vi "Rohde & Schwarz VNA Set Sweep Type.vi"(6 "Channel":i8=1 min=1 max=99 step=1, 7 "Rohde & Schwarz VNA":T1, 8 "error in (no error)":errorcluster, 10 "Sweep Type":T2, 11 "VISA Resource Name":refnum<visa-resource-name>) -> (0 "error out":errorcluster, 3 "dup VISA Resource Name":refnum<visa-resource-name>)   [LabVIEW 2011]
doc: "This VI for the HP8753B is used to set the meausurement format."
uses:
  TypeDefs/Rohde & Schwarz VNA Sweep Type.ctl
  TypeDefs/Rohde & Schwarz VNA Instrument Info.ctl
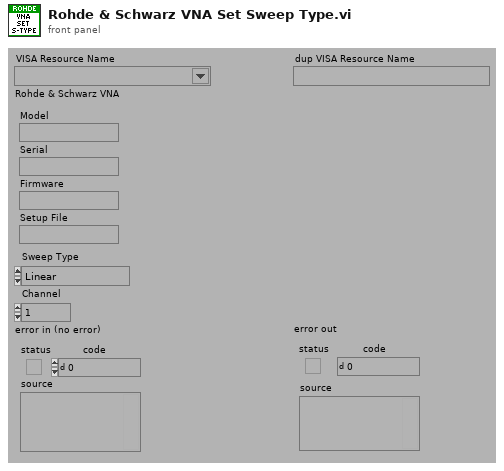
[diagram p1: front panel]
types:
  T1 = typedef "Rohde & Schwarz VNA Instrument Info.ctl" = cluster{"Model":string, "Serial":string, "Firmware":string, "Setup File":string}
  T2 = typedef "Rohde & Schwarz VNA Sweep Type.ctl" = enum32{"Linear", "Logarithmic", "Segmented", "Power", "Time", "CW"}
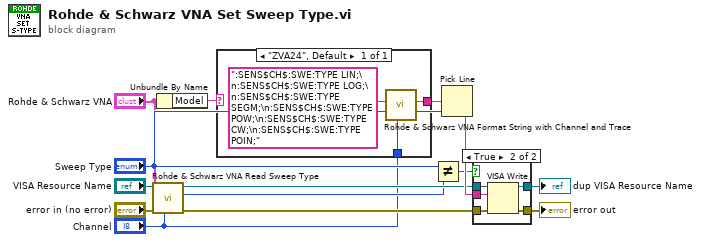
[diagram p0: block diagram]
diagram:
  n1 = call "Rohde & Schwarz VNA Read Sweep Type.vi"("Channel"="Channel", "Rohde & Schwarz VNA"="Rohde & Schwarz VNA", "error in (no error)"="error in (no error)", "VISA Resource Name"="VISA Resource Name") -> ("error out"=w9:errorcluster, "Sweep Type"=w6:T2, "dup VISA Resource Name"=w8:refnum<visa-resource-name>)  [unwired: 5 out]
  n2 = Unbundle By Name("Rohde & Schwarz VNA") -> ("Model"=w1:string)
  n3 = case shown="\"ZVA24\", Default" w1 {
    tunnel: [w16] -> w4
    tunnel: "Channel" -> [w15]
    frame "ZVA24", Default {
      n4 = call "Rohde & Schwarz VNA Format String with Channel and Trace.vi"("Channel"=w15, "String"=":SENS$CH$:SWE:TYPE LIN;\n:SENS$CH$:SWE:TYPE LOG;\n:SENS$CH$:SWE:TYPE SEGM;\n:SENS$CH$:SWE:TYPE POW;\n:SENS$CH$:SWE:TYPE CW;\n:SENS$CH$:SWE:TYPE POIN;") -> ("String Out"=w16:string)  [unwired: 1 in, 6 out]
    }
  }
  n5 = Not Equal?(x="Sweep Type", y=w6) -> (x != y?=w5:bool)
  n6 = Pick Line(multi-line string=w4, line index="Sweep Type") -> (output string=w12:string)  [unwired: 1 out]
  n7 = case shown="True" w5 {
    tunnel: [w19 w24] -> w14
    tunnel: [w18 w23] -> w13
    tunnel: w12 -> [_ w22]
    tunnel: w9 -> [w18 w21]
    tunnel: w8 -> [w19 w20]
    frame False {
    }
    frame True {
      n8 = VISA Write(VISA resource name=w20, write buffer=w22, error in (no error)=w21) -> (VISA resource name out=w24:refnum<visa-resource-name>, error out=w23:errorcluster)  [unwired: 1 out]
    }
  }
  "dup VISA Resource Name" <- w14
  "error out" <- w13
